vi "LVClass_WavefrontCorrector Get WavefrontCorrectorSet.vi"(0 "WavefrontCorrector":refnum<class "WavefrontCorrector.lvclass">, 11 "error in (no error)":errorcluster) -> (4 "WavefrontCorrector (dup)":refnum<class "WavefrontCorrector.lvclass">, 6 "WavefrontCorrectorSet":refnum<class "WavefrontCorrectorSet.lvclass">, 15 "error out":errorcluster)   [LabVIEW 2020, in "WavefrontCorrector.lvclass"]
doc: "Wavefront corrector parameter getter for parameter of type boolean.\n\n--------------------------------------------------------------------------------\n\n<B>correctorIn </B> : WavefrontCorrector object.\n<B>correctorOut </B> : WavefrontCorrector object.\n<B>parameter_name </B> : Name of the parameter.\n<B>value </B> : Value of the parameter.\n<B>ErrorIn </B> : Error\n<B>ErrorOut </B> : Error\n\n--------------------------------------------------------------------------------"
uses:
  WavefrontCorrector.lvclass
  WavefrontCorrectorSet.lvclass
  WavefrontCorrector.lvclass/WavefrontCorrector.ctl
  LVClass_WavefrontCorrectorSet Write WavefrontCorrectorSet.vi
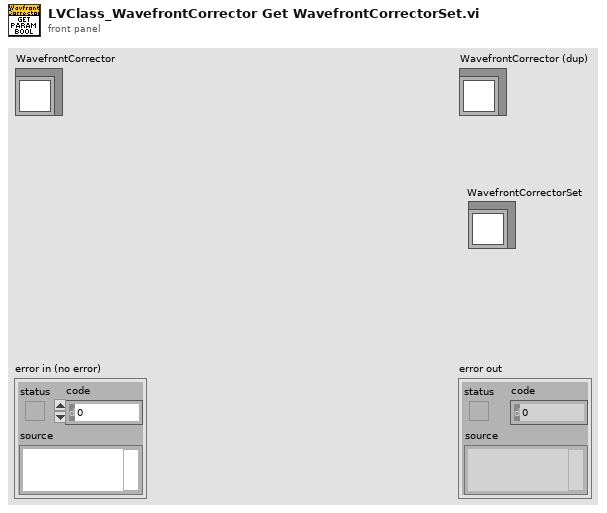
[diagram p1: front panel]
types:
  T1 = typedef "ClassID.ctl" = i64
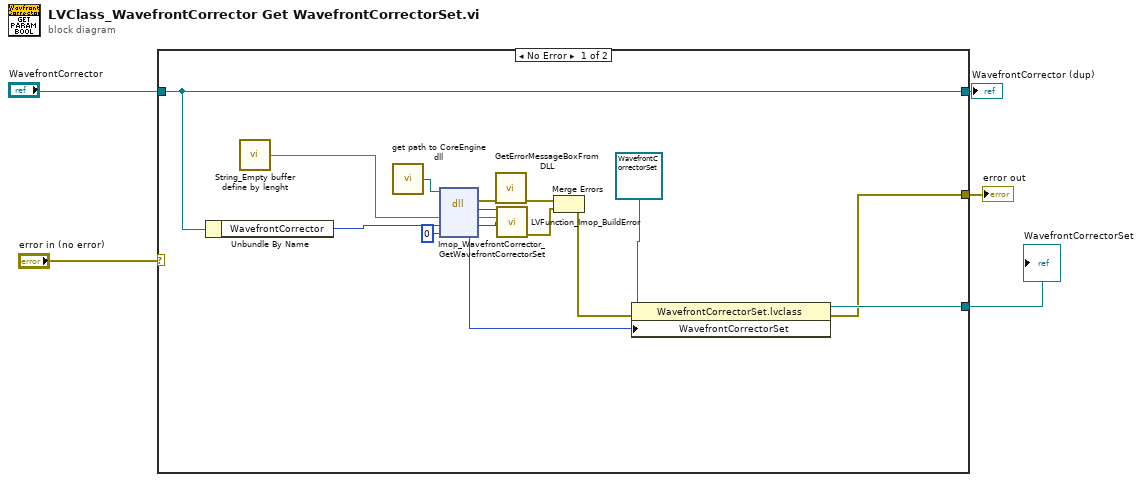
[diagram p0: block diagram]
diagram:
  n1 = case shown="No Error" "error in (no error)" {
    selector: "error in (no error)" -> [_ w23]
    tunnel: [w7 w23] -> w3
    tunnel: [w10 w22] -> w2
    tunnel: "WavefrontCorrector" -> [w10 w22]
    tunnel: [w8 _] -> w1
    frame No Error {
      n2 = Unbundle By Name(w10) -> ("WavefrontCorrector"=w20:T1)
      n3 = call "String_Empty buffer define by lenght.vi"() -> ("Empty buffer"=w21:string)  [unwired: 1 in]
      n4 = call "get path to CoreEngine dll.vi"() -> ("path to wavekit library"=w17:path)  [unwired: 14 in, 1 out]
      n5 = dll-call lib="D:/soft/HASO_v3/SVN_trunk/ImOpCoreEngine4_LV2011/DLLs/c_interface_vc100.dll" fn="Imop_WavefrontCorrector_GetWavefrontCorrectorSet"(path in=w17, "message"=w21, "camera"=w20, "CameraSet"=0) -> (error out=w16:errorcluster, "return type"=w18:i32, "message"=w19:string, "camera"=w6:i64, "CameraSet"=w12:i64)  [unwired: 2 in, 1 out]
      n6 = call "GetErrorMessageBoxFromDLL.vi"("error IN"=w16) -> ("error OUT"=w15:errorcluster)  [unwired: 10 in]
      n7 = call "LVFunction_Imop_BuildError.vi"("code"=w18, "String to Prepend to source (\"\")"=w19, "Adresse"=w6) -> ("error out"=w14:errorcluster)  [unwired: 12 in]
      n8 = Merge Errors(w15, w14) -> (w11:errorcluster)
      n9 = property class="WavefrontCorrectorSet.lvclass"(reference=refnum<class "WavefrontCorrectorSet.lvclass"> refnum ("WavefrontCorrectorSet"), error in=w11, "WavefrontCorrectorSet"=w12) -> (reference out=w8:refnum<class "WavefrontCorrectorSet.lvclass">, error out=w7:errorcluster)
    }
    frame Error {
    }
  }
  "error out" <- w3
  "WavefrontCorrector (dup)" <- w2
  "WavefrontCorrectorSet" <- w1
